vi "WaitForMessageFromAddons.vi"(8 "error in (no error)":errorcluster, 9 "timeout ms":i32=200, 10 "Name":string="Diagnostic Unlock ECU Service", 11 "TCP Ref":refnum<k5>) -> (0 "error out":errorcluster)   [LabVIEW 2019, in "Diagnostic Unlock ECU Service.lvlib"]
uses:
  Diagnostic Unlock ECU Service.lvlib
  <vilib>/NI/STM/NI STM.lvlib
  <vilib>/NI/STM/TCP/TCP Read Options.ctl
  <vilib>/Utility/SystemLogging/NI_SystemLogging.lvlib
  Service Shared/UnlockECU.SendSeedToWindowsAndWaitOnKeyCmd.ctl
  Service Shared/Diagnostic Unlock ECU Service Shared.lvlib
  Service Shared/UnlockECU.SendSeedToWindowsAndWaitOnKeyResp.ctl
  <vilib>/NI/STM/TCP/TCP Write Options.ctl
  <vilib>/NI/STM/TCP/Read Meta Data (TCP Ref).vi
  <vilib>/NI/STM/TCP/Write Message (TCP).vi
  <vilib>/NI/STM/TCP/Get Connection Reference (TCP).vi
  <vilib>/NI/STM/TCP/Read Message (TCP).vi
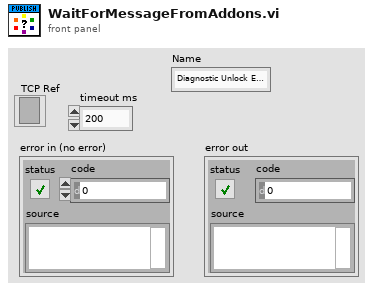
[diagram p1: front panel]
types:
  T1 = typedef "NI STM.lvlib/TCP Read Options.ctl" = cluster{"ignore timeout error":bool, "timeout ms (1000)":i32}
  T2 = typedef "NI STM.lvlib/TCP Write Options.ctl" = cluster{"ignore timeout error":bool, "timeout ms (1000)":i32}
  T3 = typedef "Diagnostic Unlock ECU Service Shared.lvlib/UnlockECU.SendSeedToWindowsAndWaitOnKeyResp.ctl" = cluster{"DLL Error":errorcluster, "Key Length":u32, "Key":u8[]}
  T4 = typedef "Diagnostic Unlock ECU Service Shared.lvlib/UnlockECU.SendSeedToWindowsAndWaitOnKeyCmd.ctl" = cluster{"Source DLL Path":path, "Security Level":u32, "Max Key Length":u32, "Seed":u8[], "ECU  Variant":i8, "Addon Name":string, "Optional Parameter":i8}
  T5 = typedef "NI STM.lvlib/TCP Connection Info.ctl" = cluster{"connection ID":refnum<k5>, "meta data":T6[]}
  T6 = typedef "NI STM.lvlib/MetaDataElement.ctl" = string
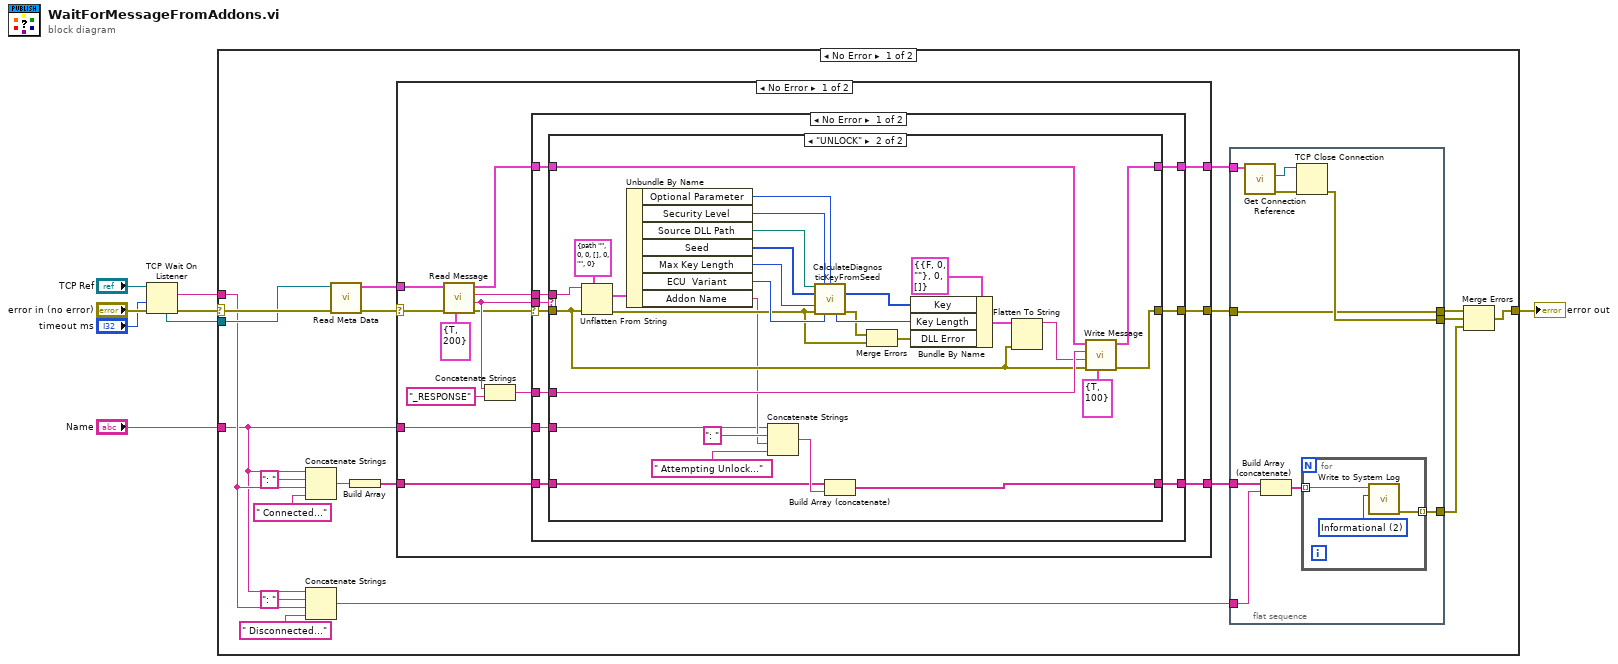
[diagram p0: block diagram]
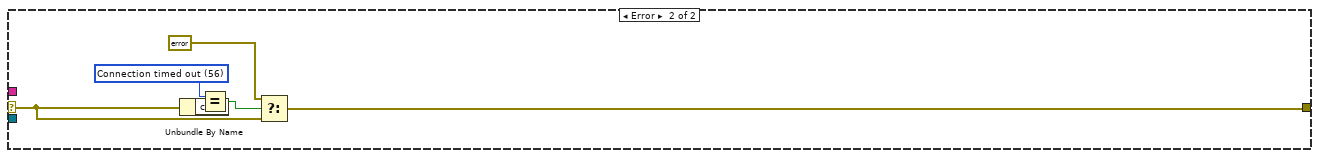
[diagram p5: hidden frame]
diagram:
  n1 = TCP Wait On Listener(8:"error in (no error)", 9:"timeout ms", 11:"TCP Ref") -> (0:w4:errorcluster, 2:w8:string, 4:w5:refnum<k5>)  [unwired: 1 in, 2 out]
  n2 = case shown="No Error" w4 {
    selector: w4 -> [w28 w105]
    tunnel: [w22 w104] -> w6
    tunnel: w5 -> [w27 _]
    tunnel: w8 -> [w11 _]
    tunnel: "Name" -> [w10 _]
    frame No Error {
      n3 = Concatenate Strings(w10, ": " ("string"), w11, " Connected..." ("string")) -> (w17:string)
      n4 = Concatenate Strings(w10, ": " ("string"), w11, " Disconnected..." ("string")) -> (w9:string)
      n5 = call-poly <vilib>:"Read Meta Data.vi"("error in"=w28, "connection ID"=w27) -> ("error out"=w25:errorcluster, "connection info out"=w26:T5)  [unwired: 7 in, 1 out]
      n6 = Build Array(w17) -> (w16:string[])
      n7 = case shown="No Error" w25 {
        selector: w25 -> [w44 w103]
        tunnel: [w46 w103] -> w20
        tunnel: w26 -> [w54 w102]
        tunnel: [w45 w102] -> w24
        tunnel: w10 -> [w43 _]
        tunnel: w16 -> [w42 w101]
        tunnel: [w41 w101] -> w15
        frame No Error {
          n8 = call-poly <vilib>:"Read Message.vi"("options"=T1 {"ignore timeout error"=TRUE, "timeout ms (1000)"=200}, "error in"=w44, "connection info in"=w54) -> ("error out"=w49:errorcluster, "name"=w51:T6, "data string"=w50:string, "connection info out"=w48:T5)  [unwired: 3 in, 2 out]
          n9 = Concatenate Strings(w51, "_RESPONSE" ("string")) -> (w47:string)
          n10 = case shown="No Error" w49 {
            selector: w49 -> [w63 w100]
            tunnel: w51 -> [w58 _]
            tunnel: w50 -> [w64 _]
            tunnel: [w62 w100] -> w46
            tunnel: w48 -> [w61 w99]
            tunnel: [w60 w99] -> w45
            tunnel: w47 -> [w59 _]
            tunnel: w43 -> [w57 _]
            tunnel: w42 -> [w56 w98]
            tunnel: [w55 w98] -> w41
            frame No Error {
              n11 = case shown="\"UNLOCK\"" w58 {
                tunnel: w64 -> [_ w97]
                tunnel: w63 -> [w67 w80]
                tunnel: [w67 w72] -> w62
                tunnel: w61 -> [w66 w94]
                tunnel: [w66 w93] -> w60
                tunnel: w59 -> [_ w92]
                tunnel: w57 -> [_ w73]
                tunnel: w56 -> [w65 w70]
                tunnel: [w65 w69] -> w55
                frame Default {
                }
                frame "UNLOCK" {
                  n12 = Unflatten From String(type=T4 {"Source DLL Path"=path "", "Security Level"=0, "Max Key Length"=0, "Seed"=[], "ECU  Variant"=0, "Addon Name"="", "Optional Parameter"=0} ("Settings"), binary string=w97, error in (no error)=w80) -> (value=w95:T4, error out=w79:errorcluster)  [unwired: 2 in, 1 out]
                  n13 = Unbundle By Name(w95) -> ("Optional Parameter"=w68:i8, "Security Level"=w87:u32, "Source DLL Path"=w91:path, "Seed"=w90:u8[], "Max Key Length"=w89:u32, "ECU  Variant"=w88:i8, "Addon Name"=w74:string)
                  n14 = Concatenate Strings(w73, ": " ("string"), w74, " Attempting Unlock..." ("string")) -> (w71:string)
                  n15 = call "CalculateDiagnosticKeyFromSeed.vi"("SeedKey DLL path"=w91, "security level"=w87, "optional parameter (OEM specific)"=w68, "seed"=w90, "maximum key length"=w89, "error in (no error)"=w79, "ECU variant"=w88) -> ("key"=w85:u8[], "key length"=w84:u32, "error out"=w78:errorcluster)  [unwired: 5 in, 1 out]
                  n16 = Build Array (concatenate)(w70, w71) -> (w69:string[])
                  n17 = Merge Errors(w78, w79) -> (w77:errorcluster)
                  n18 = Bundle By Name(cluster=T3 {"DLL Error"={"status"=FALSE, "code"=0, "source"=""}, "Key Length"=0, "Key"=[]} ("Cluster"), "Key"=w85, "Key Length"=w84, "DLL Error"=w77) -> (w83:T3)
                  n19 = Flatten To String(anything=w83, error in (no error)=w80) -> (data string=w82:string)  [unwired: 2 in, 2 out]
                  n20 = call-poly <vilib>:"Write Message.vi"("options"=T2 {"ignore timeout error"=TRUE, "timeout ms (1000)"=100}, "error in"=w80, "data"=w82, "name"=w92, "connection info in"=w94) -> ("error out"=w72:errorcluster, "connection info out"=w93:T5)  [unwired: 5 in]
                }
              }
            }
            frame Error {
            }
          }
        }
        frame Error {
        }
      }
      n21 = flat-sequence {
        tunnel: w24 -> [w36]
        tunnel: [w34] -> w23
        tunnel: [w33] -> w14
        tunnel: [w32] -> w21
        tunnel: w20 -> [w32]
        tunnel: w15 -> [w31]
        tunnel: w9 -> [w29]
        frame #0 {
          n22 = call-poly <vilib>:"Get Connection Reference.vi"("connection info in"=w36) -> ("error out"=w35:errorcluster, "connection ID out"=w37:refnum<k5>)  [unwired: 8 in, 1 out]
          n23 = Build Array (concatenate)(w31, w29) -> (w30:string[])
          n24 = TCP Close Connection(connection ID=w37, error in (no error)=w35) -> (error out=w34:errorcluster)  [unwired: 1 in, 1 out]
          n25 = for {
            tunnel: w30 -> [w39] mode=indexing
            tunnel: [w38] -> w33 mode=indexing
            w40 = 2 items=["Error", "Warning", "Informational"] ("severity")
            n26 = call <vilib>:"Write to System Log.vi"("severity"=w40, "message"=w39) -> ("error out"=w38:errorcluster)  [unwired: 9 in]
          }
        }
      }
      n27 = Merge Errors(w21, w23, w14) -> (w22:errorcluster)
    }
    frame Error {
      w106 = 56 items=["No Error", "Argument Error", "Memory Full", "Out of Zone", "End of File", "File Already Open", "Generic File IO Error", "File Not Found", "File Permission Error", "Disk Full", "Duplicate Path", "Too Many Files Open", "Not Enabled", "Resource File Not Found", "Cannot Add Resource", "Resource Not Found", "Image Not Found", "Image Memory Error", "Pen Does Not Exist", "Config Bad Type", "Config Token Not Found", "Config Parse Error", "Config Memory Error", "Bad External Code Format", "Bad External Code Offset", "External Code Not Present", "Null Window", "Destroy Window Mixup", "Null Menu", "Print Aborted", "Bad Print Record", "Print Driver Error", "Windows Error During Print", "Memory Error During Print", "Print Dialog Error", "Generic Print Error", "Invalid Device Refnum", "Device Not Found", "Device Parameter Error", "Device Unit Error", "Can't Open Device", "Device Call Aborted", "Generic Error", "Cancelled By User", "Object ID Too Low", "Object ID Too High", "Object Not In Heap", "Unknown Heap", "Bad DefProc ID", "DefProc Not In Table", "Message Out Of Range", "Null Method", "Unknown Message", "Manager Call Not Supported", "Bad address", "Connection In progress", "Connection timed out", "Connection is already in progress", "Network attribute not supported", "Network error", "Address in use", "System out of memory", "Connection aborted", "Connection refused", "Connection is not connected", "Connection is already connected", "Connection closed", "Initialize error (interapplication manager)", "Bad occurrence", "Wait on unbound occurrence handler", "Occurrence queue overflow", "Bad path", "Semaphore not signaled", "Unrecognized type (interapplication manager)"] ("1st Error to Convert")
      n28 = Unbundle By Name(w105) -> ("code"=w108:i32)
      n29 = Equal?(x=w106, y=w108) -> (x = y?=w109:bool)
      n30 = Select(t=errorcluster {"status"=FALSE, "code"=0, "source"=""} ("error in (no error)"), s=w109, f=w105) -> (s? t:f=w104:errorcluster)
    }
  }
  "error out" <- w6
